vi "VI Tree.vi"   [LabVIEW 2023, in "Keysight-33500B.lvlib"]
doc: "This is the instrument driver for the Agilent 3352X. It includes 33500 series models and 33600 series models. The VI Tree displays all the user-callable VIs of the instrument driver in an organized table."
uses:
  Keysight-33500B.lvlib
  Configure/Configure Standard Waveform Advanced (Pulse).vi
  Configure/Modulation/Configure Modulation (Amplitude).vi
panel:
  # "(c) 2011 - 2019 National Instruments.  ALL RIGHTS RESERVED."
  # "SEE DIAGRAM\nFOR VI TREE."
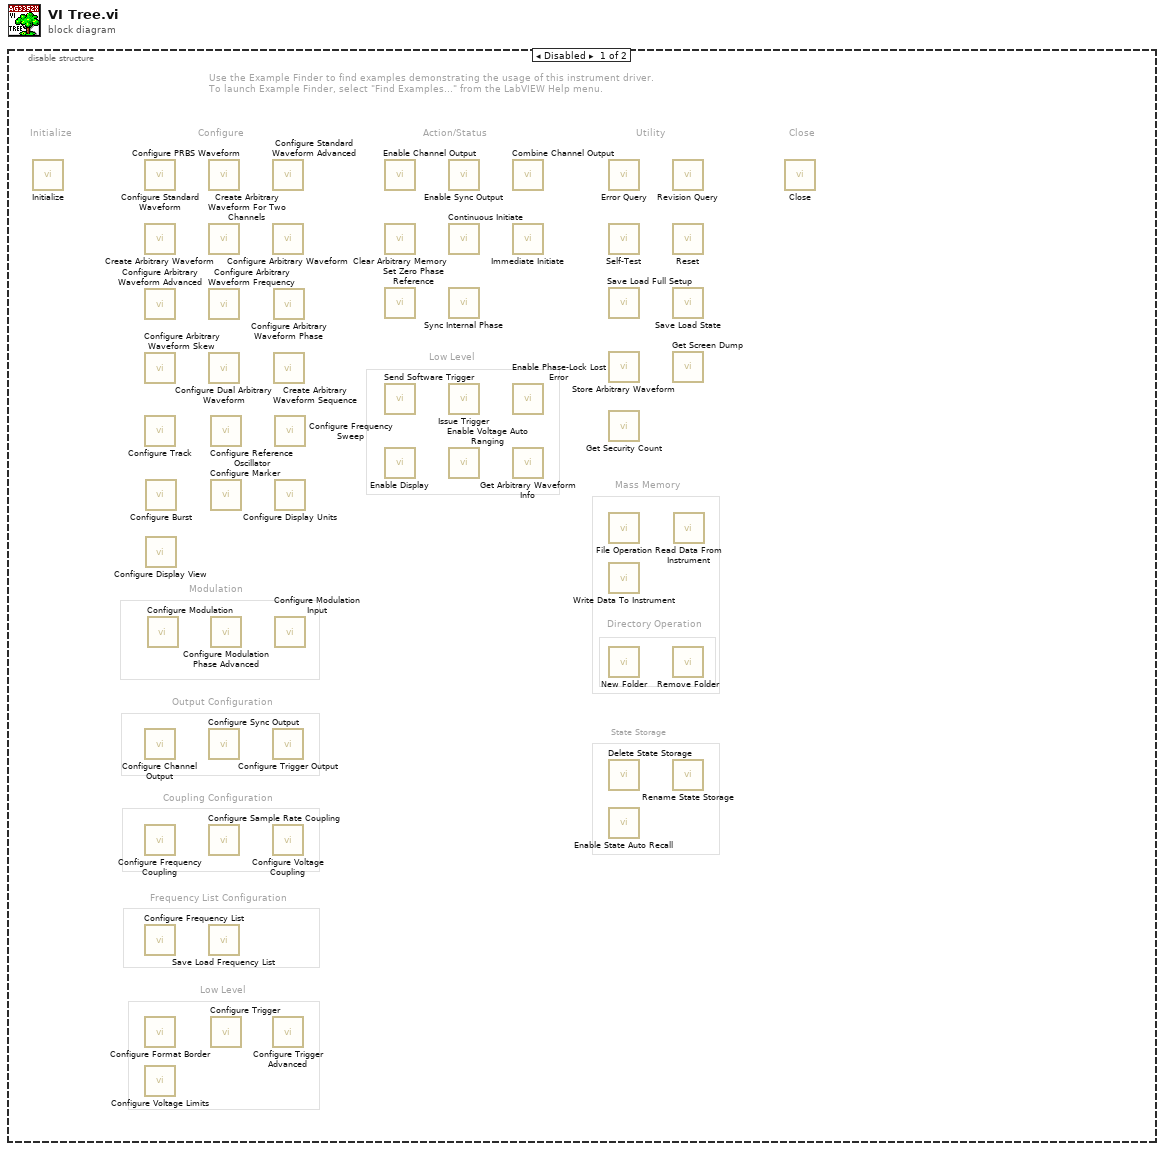
[diagram p0: block diagram]
diagram:
  n1 = disable-structure shown="Disabled" {
    frame Disabled {
      # "Directory Operation"
      # "State Storage"
      # "Mass Memory"
      # "Frequency List Configuration"
      # "Coupling Configuration"
      # "Output Configuration"
      # "Modulation"
      # "Low Level"
      # "Low Level"
      # "Use the Example Finder to find examples demonstrating the usage of this instrument driver.\nTo launch Example Finder, select \"Find Examples...\" from the LabVIEW Help menu."
      # "Configure"
      # "Utility"
      # "Action/Status"
      # "Close"
      # "Initialize"
      n2 = call "Initialize.vi"() -> ()  [unwired: 10 in, 2 out]
      n3 = call "Configure Standard Waveform.vi"() -> ()  [unwired: 14 in, 2 out]
      n4 = call "Create Arbitrary Waveform.vi"() -> ()  [unwired: 10 in, 2 out]
      n5 = call "Configure Arbitrary Waveform Advanced.vi"() -> ()  [unwired: 10 in, 2 out]
      n6 = call "Configure Arbitrary Waveform Skew.vi"() -> ()  [unwired: 10 in, 2 out]
      n7 = call "Configure Track.vi"() -> ()  [unwired: 10 in, 2 out]
      n8 = call "Configure Channel Output.vi"() -> ()  [unwired: 14 in, 2 out]
      n9 = call "Configure Frequency Coupling.vi"() -> ()  [unwired: 10 in, 2 out]
      n10 = call "Configure Frequency List.vi"() -> ()  [unwired: 10 in, 2 out]
      n11 = call "Configure Format Border.vi"() -> ()  [unwired: 10 in, 2 out]
      n12 = call "Configure Voltage Limits.vi"() -> ()  [unwired: 10 in, 2 out]
      n13 = call "Configure Burst.vi"() -> ()  [unwired: 14 in, 2 out]
      n14 = call "Configure Display View.vi"() -> ()  [unwired: 10 in, 2 out]
      n15 = call-poly "Configure Modulation.vi"() -> ()  [unwired: 14 in, 2 out]
      n16 = call "Configure PRBS Waveform.vi"() -> ()  [unwired: 10 in, 2 out]
      n17 = call "Create Arbitrary Waveform For Two Channels.vi"() -> ()  [unwired: 10 in, 2 out]
      n18 = call "Configure Arbitrary Waveform Frequency.vi"() -> ()  [unwired: 10 in, 2 out]
      n19 = call "Configure Dual Arbitrary Waveform.vi"() -> ()  [unwired: 10 in, 2 out]
      n20 = call "Configure Sync Output.vi"() -> ()  [unwired: 10 in, 2 out]
      n21 = call "Configure Sample Rate Coupling.vi"() -> ()  [unwired: 14 in, 2 out]
      n22 = call "Save Load Frequency List.vi"() -> ()  [unwired: 10 in, 2 out]
      n23 = call "Configure Reference Oscillator.vi"() -> ()  [unwired: 10 in, 2 out]
      n24 = call "Configure Marker.vi"() -> ()  [unwired: 10 in, 2 out]
      n25 = call "Configure Modulation Phase Advanced.vi"() -> ()  [unwired: 10 in, 2 out]
      n26 = call "Configure Trigger.vi"() -> ()  [unwired: 10 in, 2 out]
      n27 = call-poly "Configure Standard Waveform Advanced.vi"() -> ()  [unwired: 10 in, 2 out]
      n28 = call "Configure Arbitrary Waveform.vi"() -> ()  [unwired: 14 in, 2 out]
      n29 = call "Configure Trigger Output.vi"() -> ()  [unwired: 10 in, 2 out]
      n30 = call "Configure Voltage Coupling.vi"() -> ()  [unwired: 10 in, 2 out]
      n31 = call "Configure Trigger Advanced.vi"() -> ()  [unwired: 10 in, 2 out]
      n32 = call "Configure Arbitrary Waveform Phase.vi"() -> ()  [unwired: 10 in, 2 out]
      n33 = call "Create Arbitrary Waveform Sequence.vi"() -> ()  [unwired: 10 in, 2 out]
      n34 = call "Configure Frequency Sweep.vi"() -> ()  [unwired: 14 in, 2 out]
      n35 = call "Configure Display Units.vi"() -> ()  [unwired: 10 in, 2 out]
      n36 = call "Configure Modulation Input.vi"() -> ()  [unwired: 10 in, 2 out]
      n37 = call "Enable Channel Output.vi"() -> ()  [unwired: 10 in, 2 out]
      n38 = call "Clear Arbitrary Memory.vi"() -> ()  [unwired: 10 in, 2 out]
      n39 = call "Set Zero Phase Reference.vi"() -> ()  [unwired: 10 in, 2 out]
      n40 = call "Send Software Trigger.vi"() -> ()  [unwired: 10 in, 2 out]
      n41 = call "Enable Display.vi"() -> ()  [unwired: 10 in, 2 out]
      n42 = call "Enable Sync Output.vi"() -> ()  [unwired: 10 in, 2 out]
      n43 = call "Continuous Initiate.vi"() -> ()  [unwired: 10 in, 2 out]
      n44 = call "Sync Internal Phase.vi"() -> ()  [unwired: 10 in, 2 out]
      n45 = call "Issue Trigger.vi"() -> ()  [unwired: 10 in, 2 out]
      n46 = call "Enable Voltage Auto Ranging.vi"() -> ()  [unwired: 10 in, 2 out]
      n47 = call "Combine Channel Output.vi"() -> ()  [unwired: 10 in, 2 out]
      n48 = call "Immediate Initiate.vi"() -> ()  [unwired: 10 in, 2 out]
      n49 = call "Enable Phase-Lock Lost Error.vi"() -> ()  [unwired: 10 in, 2 out]
      n50 = call "Get Arbitrary Waveform Info.vi"() -> ()  [unwired: 9 in, 3 out]
      n51 = call "Error Query.vi"() -> ()  [unwired: 8 in, 4 out]
      n52 = call "Self-Test.vi"() -> ()  [unwired: 8 in, 4 out]
      n53 = call "Save Load Full Setup.vi"() -> ()  [unwired: 10 in, 2 out]
      n54 = call "Store Arbitrary Waveform.vi"() -> ()  [unwired: 10 in, 2 out]
      n55 = call "Get Security Count.vi"() -> ()  [unwired: 9 in, 3 out]
      n56 = call "File Operation.vi"() -> ()  [unwired: 10 in, 2 out]
      n57 = call "Write Data To Instrument.vi"() -> ()  [unwired: 10 in, 2 out]
      n58 = call "New Folder.vi"() -> ()  [unwired: 10 in, 2 out]
      n59 = call "Delete State Storage.vi"() -> ()  [unwired: 10 in, 2 out]
      n60 = call "Enable State Auto Recall.vi"() -> ()  [unwired: 10 in, 2 out]
      n61 = call "Revision Query.vi"() -> ()  [unwired: 8 in, 4 out]
      n62 = call "Reset.vi"() -> ()  [unwired: 10 in, 2 out]
      n63 = call "Save Load State.vi"() -> ()  [unwired: 10 in, 2 out]
      n64 = call "Get Screen Dump.vi"() -> ()  [unwired: 10 in, 2 out]
      n65 = call "Remove Folder.vi"() -> ()  [unwired: 10 in, 2 out]
      n66 = call "Rename State Storage.vi"() -> ()  [unwired: 10 in, 2 out]
      n67 = call "Read Data From Instrument.vi"() -> ()  [unwired: 9 in, 3 out]
      n68 = call "Close.vi"() -> ()  [unwired: 11 in, 1 out]
    }
    frame Enabled {
    }
  }
